vi "MatrixUtil_Zero.vi"(11 "input matrix":T1) -> (3 "output matrix":T1)   [LabVIEW 2019, in "Trajectory_Library.lvlib"]
doc: "Creates a new LINEAR SYSTEM data cluster with the specified values. \n\n\nInputs: \n - XXX -- XXX.\n\nOutputs:\n - XXX -- XXX."
uses:
  Trajectory_Library.lvlib
  <vilib>/Analysis/Matrix/Datatypes/RealMatrix.ctl
  <vilib>/Analysis/Matrix/NI_Matrix.lvlib
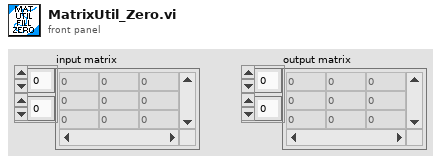
[diagram p1: front panel]
types:
  T1 = typedef "NI_Matrix.lvlib/RealMatrix.ctl" = dbl[][]
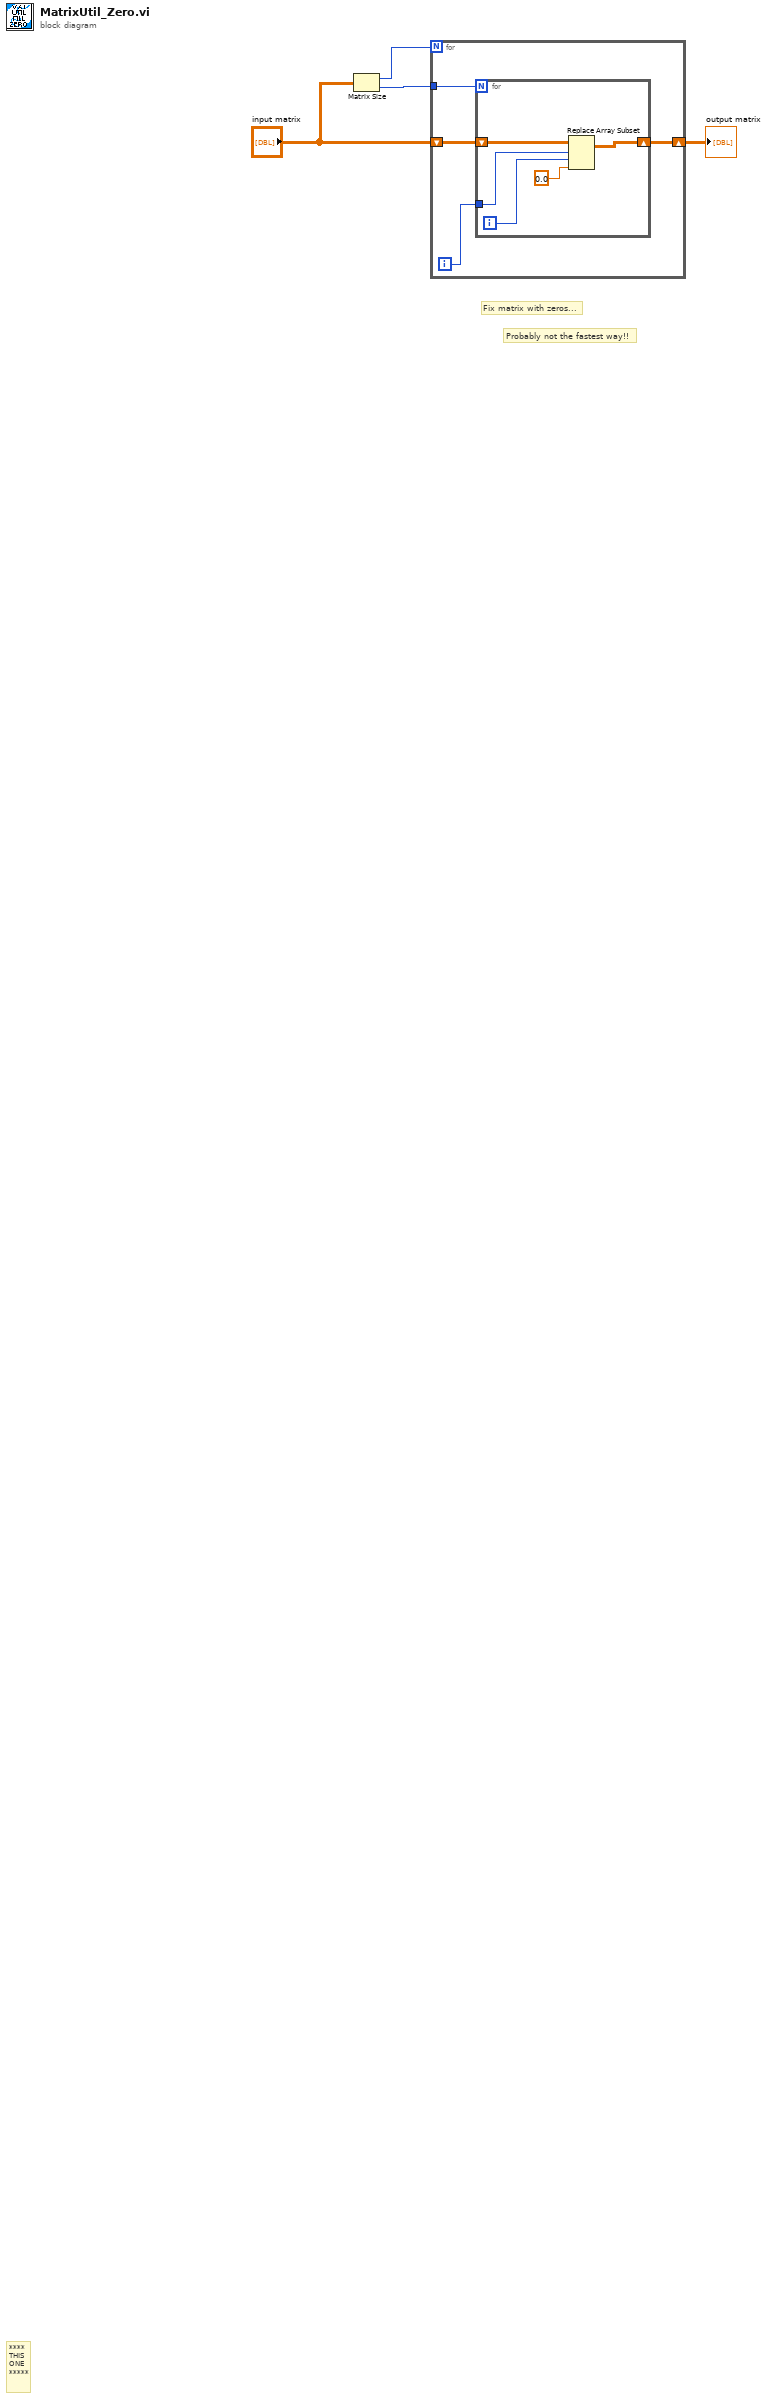
[diagram p0: block diagram]
diagram:
  # "Probably not the fastest way!!"
  # "Fix matrix with zeros..."
  # "****\nTHIS\nONE\n*****"
  n1 = Matrix Size(0:"input matrix") -> (1:w3:i32, 2:w2:i32)
  n2 = for {
    N: w3 -> [_]
    shift-right: [w5] -> w1
    shift-left: "input matrix" -> [w8]
    tunnel: w2 -> [w6]
    i -> [w7]
    n3 = for {
      N: w6 -> [_]
      shift-right: [w9] -> w5
      shift-left: w8 -> [w13]
      tunnel: w7 -> [w10]
      i -> [w11]
      n4 = Replace Array Subset(array=w13, new element=0.0 ("new element/submatrix"), index (row)=w10, index (col)=w11) -> (w9:T1)
    }
  }
  "output matrix" <- w1
